vi "FailureDescription.vi"(8 "error in (no error)":errorcluster, 10 "Actual":variant, 11 "Binary Operator in":refnum<class "Binary Operator.lvclass">) -> (0 "error out":errorcluster, 2 "Failure Description":string, 3 "Binary Operator out":refnum<class "Binary Operator.lvclass">)   [LabVIEW 2017, in "Transparent Assertions.lvlib" / "Constraints.lvlib" / "Binary Operator.lvclass"]
doc: "Return the second part of the scentence \"Failed asserting that ...\""
uses:
  Binary Operator.lvclass
  Binary Operator.lvclass/Binary Operator.ctl
  Constraint/Constraint.lvclass
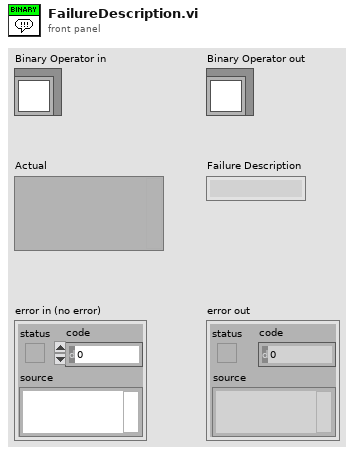
[diagram p1: front panel]
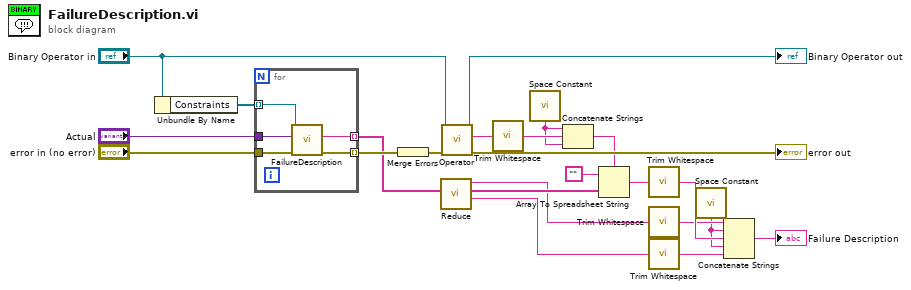
[diagram p0: block diagram]
diagram:
  n1 = Unbundle By Name("Binary Operator in") -> ("Constraints"=w21:refnum<class "Constraint.lvclass">[])
  n2 = for {
    tunnel: w21 -> [w26] mode=indexing
    tunnel: "error in (no error)" -> [w28]
    tunnel: [w27] -> w22 mode=indexing
    tunnel: [w25] -> w9 mode=indexing
    tunnel: "Actual" -> [w24]
    n3 = call-dynamic "FailureDescription.vi"("error in (no error)"=w28, "Actual"=w24, "Constraint in"=w26) -> ("error out"=w27:errorcluster, "Failure Description"=w25:string)  [unwired: 6 in, 1 out]
  }
  n4 = Merge Errors(w22) -> (w19:errorcluster)
  n5 = call "Reduce.vi"("Failure Descriptions"=w9) -> ("Suffix"=w2:string, "Failure Descriptions out"=w8:string[], "Prefix"=w6:string)  [unwired: 8 in]
  n6 = call-dynamic "Operator.vi"("error in (no error)"=w19, "Binary Operator in"="Binary Operator in") -> ("error out"=→"error out":errorcluster, "Operator"=w15:string, "Binary Operator out"=→"Binary Operator out":refnum<class "Binary Operator.lvclass">)  [unwired: 7 in]
  n7 = call <vilib>:"Trim Whitespace.vi"("string"=w15) -> ("trimmed string"=w13:string)  [unwired: 1 in]
  n8 = call <vilib>:"Space Constant.vi"() -> ("String"=w12:string)
  n9 = Concatenate Strings(w12, w13, w12) -> (w14:string)
  n10 = Array To Spreadsheet String(delimiter (Tab)=w14, array=w8, 3:"") -> (spreadsheet string=w11:string)
  n11 = call <vilib>:"Trim Whitespace.vi"("string"=w11) -> ("trimmed string"=w7:string)  [unwired: 1 in]
  n12 = call <vilib>:"Trim Whitespace.vi"("string"=w6) -> ("trimmed string"=w5:string)  [unwired: 1 in]
  n13 = call <vilib>:"Trim Whitespace.vi"("string"=w2) -> ("trimmed string"=w1:string)  [unwired: 1 in]
  n14 = call <vilib>:"Space Constant.vi"() -> ("String"=w3:string)
  n15 = Concatenate Strings(w5, w3, w7, w3, w1) -> (→"Failure Description":string)
